vi "Get All Items.vi"(7 "Calling VI Ref":refnum<vi>, 8 "error in (no error)":errorcluster, 11 "Path":path) -> (0 "error out":errorcluster, 2 "Cancelled?":bool, 3 "Item Data":refnum<class "Item.lvclass">[](array[class]))   [LabVIEW 2020, in "VI Properties Editor.lvlib"]
doc: "Gets all VI data from the source of VIs located at <B>Path</B>."
uses:
  VI Properties Editor.lvlib
  Classes/Item/Item.lvclass
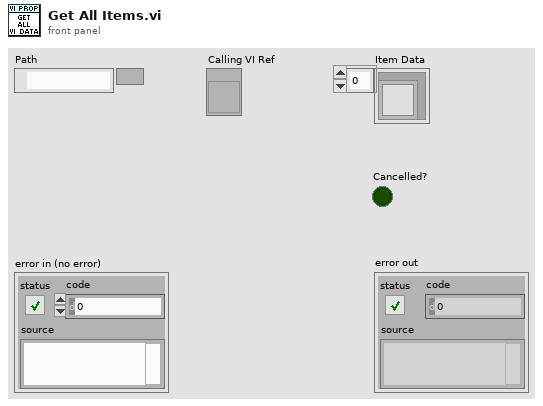
[diagram p1: front panel]
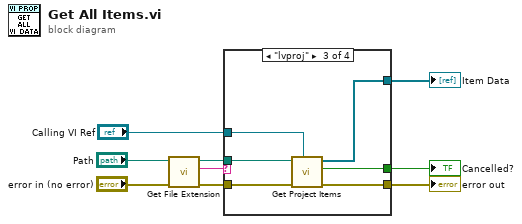
[diagram p0: block diagram]
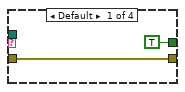
[diagram p2: hidden frame]
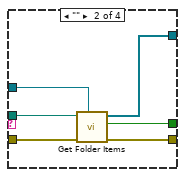
[diagram p3: hidden frame]
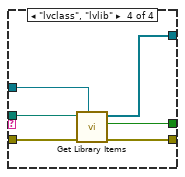
[diagram p4: hidden frame]
diagram:
  n1 = call <vilib>:"Get File Extension.vi"("error in (no error)"="error in (no error)", "file"="Path") -> ("error out"=w5:errorcluster, "lowercase file extension"=w7:string, "dup file"=w6:path)  [unwired: 5 in, 2 out]
  n2 = case shown="\"lvproj\"" w7 {
    tunnel: w6 -> [_ w16 w22 w28]
    tunnel: w5 -> [w11 w17 w23 w29]
    tunnel: [w11 w15 w21 w27] -> w4
    tunnel: [_ w14 w20 w26] -> w3
    tunnel: "Calling VI Ref" -> [_ w13 w19 w25]
    tunnel: [TRUE ("Cancelled?") w12 w18 w24] -> w1
    frame Default {
    }
    frame "" {
      n3 = call "Get Folder Items.vi"("Calling VI Ref"=w13, "error in (no error)"=w17, "Folder Path"=w16) -> ("error out"=w15:errorcluster, "Cancelled?"=w12:bool, "Item Data"=w14:refnum<class "Item.lvclass">[])  [unwired: 6 in]
    }
    frame "lvproj" {
      n4 = call "Get Project Items.vi"("Calling VI Ref"=w19, "error in (no error)"=w23, "Path"=w22) -> ("error out"=w21:errorcluster, "Cancelled?"=w18:bool, "Items Data"=w20:refnum<class "Item.lvclass">[])  [unwired: 6 in]
    }
    frame "lvclass", "lvlib" {
      n5 = call "Get Library Items.vi"("Calling VI Ref"=w25, "error in (no error)"=w29, "Path"=w28) -> ("error out"=w27:errorcluster, "Cancelled?"=w24:bool, "Items Data"=w26:refnum<class "Item.lvclass">[])  [unwired: 6 in]
    }
  }
  "error out" <- w4
  "Item Data" <- w3
  "Cancelled?" <- w1
